vi "1WIRE_ReadBit_multi.vi"(8 "error in":errorcluster) -> (0 "error out":errorcluster, 2 "Bit Read":bool)   [LabVIEW 2016]
doc: "This VI is created by Vincent Claes for FPDA-1 more information on http://pwo.fpga.be\n\nvincent.claes@xios.be\nclaesvincent@gmail.com\n\nhttp://www.linkedin.com/in/vincentclaes"
uses:
  <vilib>/rvi/eio/common/nirviEmuTemplateMethod_errors.vi
  <vilib>/eio/EIONode/EIONode.xnode
  <vilib>/eio/EIOMethodNode/EIOMethodNode.xnode
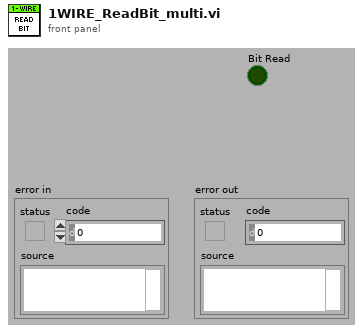
[diagram p1: front panel]
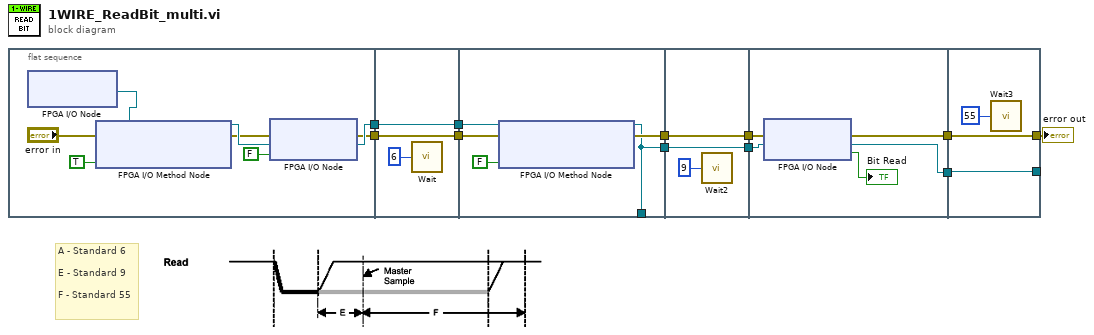
[diagram p0: block diagram]
diagram:
  # "A - Standard 6\n\nE - Standard 9\n\nF - Standard 55"
  n1 = flat-sequence {
    tunnel: [w17] -> w11
    tunnel: [w16] -> w5
    tunnel: w11 -> [w21]
    tunnel: [w21] -> w10
    tunnel: w5 -> [w20]
    tunnel: [w20] -> w4
    tunnel: w10 -> [w27]
    tunnel: [w24] -> w8
    tunnel: [w26] -> w6
    tunnel: w4 -> [w25]
    tunnel: [w24] -> _
    tunnel: [w29] -> w9
    tunnel: w8 -> [w29]
    tunnel: [w28] -> w7
    tunnel: w6 -> [w28]
    tunnel: w9 -> [w34]
    tunnel: w7 -> [w33]
    tunnel: [w32] -> w3
    tunnel: [w31] -> w1
    tunnel: [w37] -> w2
    tunnel: w3 -> [w37]
    tunnel: [w36] -> _
    tunnel: w1 -> [w36]
    frame #0 {
      n2 = xnode "FPGA I/O Node"() -> ("FPGA I/O Out"=w12:refnum<k21>)  [unwired: 1 in, 1 out]
      n3 = xnode "FPGA I/O Method Node"("error in"="error in", "FPGA I/O In"=w12, "Enable"=TRUE) -> ("error out"=w15:errorcluster, "FPGA I/O Out"=w18:refnum<k21>)
      n4 = xnode "FPGA I/O Node"("error in"=w15, "I/O Item"=FALSE ("FX2_IO1_J1_0"), "FPGA I/O In"=w18) -> ("error out"=w16:errorcluster, "FPGA I/O Out"=w17:refnum<k21>)
    }
    frame #1 {
      n5 = call "Wait"("Count(uSec)"=u32 6) -> ()  [unwired: 1 out]
    }
    frame #2 {
      n6 = xnode "FPGA I/O Method Node"("error in"=w25, "FPGA I/O In"=w27, "Enable"=FALSE) -> ("error out"=w26:errorcluster, "FPGA I/O Out"=w24:refnum<k21>)
    }
    frame #3 {
      n7 = call "Wait2"("Count(uSec)"=u32 9) -> ()  [unwired: 1 out]
    }
    frame #4 {
      n8 = xnode "FPGA I/O Node"("error in"=w33, "FPGA I/O In"=w34) -> ("error out"=w32:errorcluster, "I/O Item"=→"Bit Read":bool, "FPGA I/O Out"=w31:refnum<k21>)
    }
    frame #5 {
      n9 = call "Wait3"("Count(uSec)"=u32 55) -> ()  [unwired: 1 out]
    }
  }
  "error out" <- w2
